vi "close.vi"(8 "error in (no error)":errorcluster, 11 "TCPConnection in":refnum<class "TCPConnection.lvclass">) -> (0 "error out":errorcluster, 3 "TCPConnection out":refnum<class "TCPConnection.lvclass">)   [LabVIEW 2023, in "TCPConnection.lvclass"]
uses:
  TCPConnection.lvclass
  TCPConnection.lvclass/TCPConnection.ctl
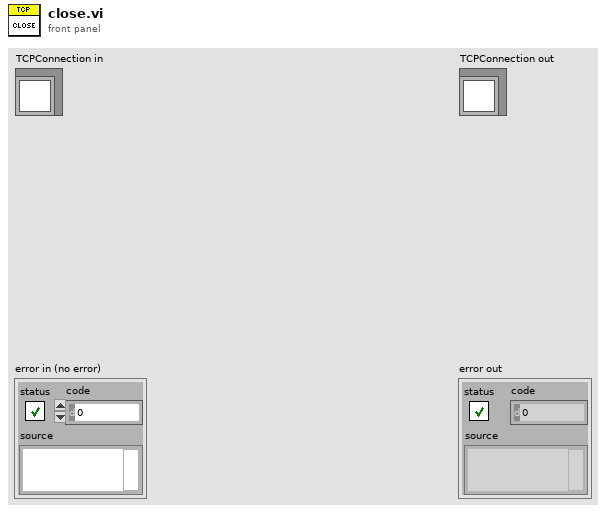
[diagram p1: front panel]
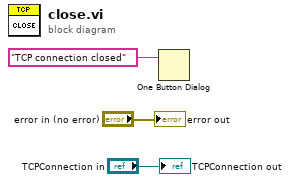
[diagram p0: block diagram]
diagram:
  n1 = One Button Dialog(message="TCP connection closed") -> ()  [unwired: 1 in, 1 out]
  "error out" <- "error in (no error)"
  "TCPConnection out" <- "TCPConnection in"
